vi "Create Name List.vi"(0 "# of Elements":i32, 7 "Prefix":string) -> (4 "Output Array":string[](array[string]))   [LabVIEW 2016]
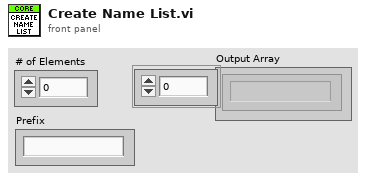
[diagram p1: front panel]
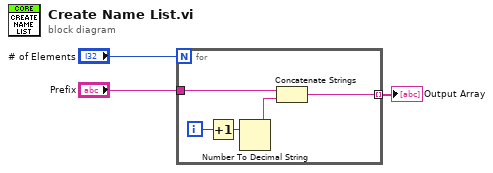
[diagram p0: block diagram]
diagram:
  n1 = for {
    N: "# of Elements" -> [_]
    tunnel: "Prefix" -> [w8]
    tunnel: [w4] -> w1 mode=indexing
    i -> [w7]
    n2 = Increment(x=w7) -> (x+1=w6:i32)
    n3 = Number To Decimal String(number=w6) -> (decimal integer string=w5:string)  [unwired: 1 in]
    n4 = Concatenate Strings(w8, w5) -> (w4:string)
  }
  "Output Array" <- w1
